vi "4461 Autophase.vi"(8 "error in (no error)":errorcluster, 10 "Results":T1, 11 "Lockin.DAQ in":refnum<class "Lockin.DAQ.lvclass">) -> (0 "error out":errorcluster, 3 "Lockin.DAQ out":refnum<class "Lockin.DAQ.lvclass">)   [LabVIEW 2016, in "Lockin.DAQ.lvclass"]
uses:
  Lockin.DAQ.lvclass
  Typedefs/Results--Cluster.ctl
  Lockin.DAQ.lvclass/Lockin.DAQ.ctl
panel:
  in  "D":dbl=0.019999999999999997 format="%.2f"
  in  "I":dbl=0.6 format="%.2f"
  in  "P":dbl=0.5 format="%.2f"
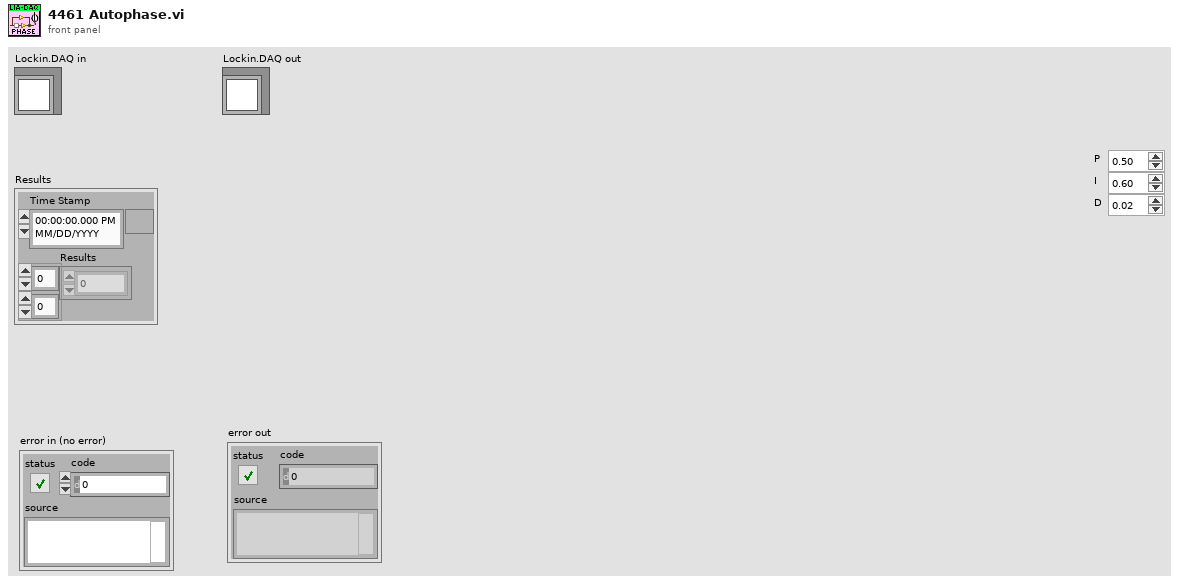
[diagram p1: front panel]
types:
  T1 = typedef "Lockin.DAQ.lvclass/Results--Cluster.ctl" = cluster{"Time Stamp":timestamp, "Results":dbl[][]}
  T2 = typedef "Lockin.DAQ.lvclass/REF-cluster.ctl" = T3[]
  T3 = typedef "Instrument.Lockin.UI.lvclass/REF Channel--Cluster.ctl" = cluster{"Enable?":bool, "Channel":i32, "Frequency":dbl, "Phase":dbl, "TC":dbl, "Order":i32}
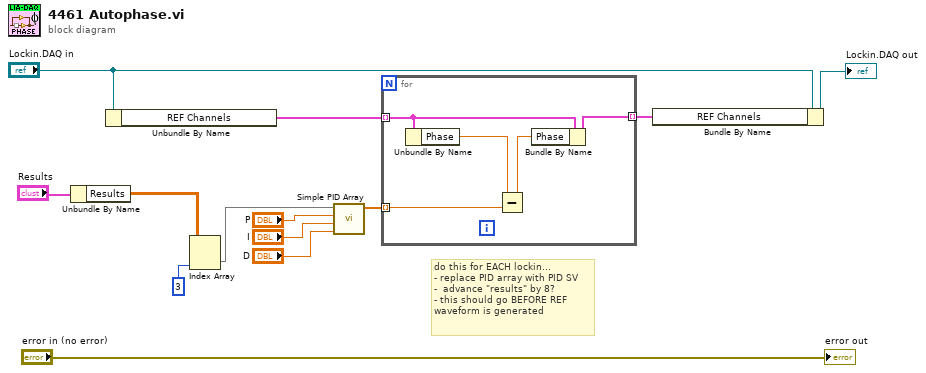
[diagram p0: block diagram]
diagram:
  # "do this for EACH lockin...\n- replace PID array with PID SV\n-  advance \"results\" by 8?\n- this should go BEFORE REF\nwaveform is generated"
  n1 = Unbundle By Name("Results") -> ("Results"=w5:dbl[][])
  n2 = Unbundle By Name("Lockin.DAQ in") -> ("REF Channels"=w2:T2)
  n3 = Index Array(array=w5, index (col)=3 ("index (row)")) -> (element=w8:dbl[])  [unwired: 1 in]
  n4 = call "Simple PID Array.vi"("D"="D", "I"="I", "P"="P", "process variable"=w8) -> ("output value"=w12:dbl[])  [unwired: 7 in]
  n5 = for {
    tunnel: w12 -> [w18] mode=indexing
    tunnel: w2 -> [w16] mode=indexing
    tunnel: [w14] -> w1 mode=indexing
    n6 = Unbundle By Name(w16) -> ("Phase"=w17:dbl)
    n7 = Subtract(x=w17, y=w18) -> (x-y=w15:dbl)
    n8 = Bundle By Name(cluster=w16, "Phase"=w15) -> (w14:T3)
  }
  n9 = Bundle By Name(cluster="Lockin.DAQ in", "REF Channels"=w1) -> (→"Lockin.DAQ out":refnum<class "Lockin.DAQ.lvclass">)
  "error out" <- "error in (no error)"
